vi "zmq_getsocketopt_binary.vi"(3 "error in":errorcluster, 4 "option":T1, 5 "socket in":refnum<class "Socket.lvclass">) -> (0 "error out":errorcluster, 1 "value":string, 2 "socket out":refnum<class "Socket.lvclass">)   [LabVIEW 2025, in "ZeroMQ.lvlib" / "Socket.lvclass"]
doc: "Query the value of <b>option</b> for the given <b>socket</b>.\n\nYou are responsible for selecting the correct polymorphic instance for the option you wish to query. Valid options of the binary type are: ZMQ_IDENTITY\n\nFurther API documentation: http://api.zeromq.org/3-2:zmq-getsockopt"
uses:
  Socket.lvclass
  socket_options.ctl
  Socket.lvclass/Socket.ctl
  ZeroMQ.lvlib
panel:
  out "len":u32
  # "ØMQ"
  # "labview"
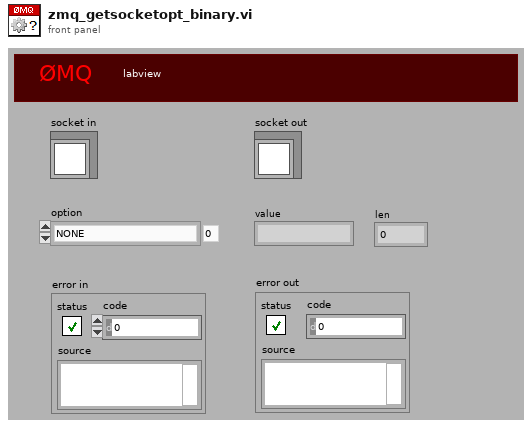
[diagram p1: front panel]
types:
  T1 = typedef "ZeroMQ.lvlib/socket_options.ctl" = enum8{"NONE", "ZMQ_HWM", "<2>", "ZMQ_SWAP", "ZMQ_AFFINITY", "ZMQ_ROUTING_ID", "ZMQ_SUBSCRIBE", "ZMQ_UNSUBSCRIBE", "ZMQ_RATE", "ZMQ_RECOVERY_IVL", "ZMQ_MCAST_LOOP", "ZMQ_SNDBUF", "ZMQ_RCVBUF", "ZMQ_RCVMORE", "ZMQ_FD", "ZMQ_EVENTS", "ZMQ_TYPE", "ZMQ_LINGER", "ZMQ_RECONNECT_IVL", "ZMQ_BACKLOG", "ZMQ_RECOVERY_IVL_MSEC", "ZMQ_RECONNECT_IVL_MAX", "ZMQ_MAXMSGSIZE", "ZMQ_SNDHWM", "ZMQ_RCVHWM", "ZMQ_MULTICAST_HOPS", "<26>", "ZMQ_RCVTIMEO", "ZMQ_SNDTIMEO", "<29>", "<30>", "ZMQ_IPV4ONLY", "ZMQ_LAST_ENDPOINT", "ZMQ_ROUTER_MANDATORY", "ZMQ_TCP_KEEPALIVE", "ZMQ_TCP_KEEPALIVE_CNT", "ZMQ_TCP_KEEPALIVE_IDLE", "ZMQ_TCP_KEEPALIVE_INTVL", "ZMQ_TCP_ACCEPT_FILTER", "ZMQ_IMMEDIATE", "ZMQ_XPUB_VERBOSE", "ZMQ_ROUTER_RAW", "ZMQ_IPV6", "ZMQ_MECHANISM", "ZMQ_PLAIN_SERVER", "ZMQ_PLAIN_USERNAME", "ZMQ_PLAIN_PASSWORD", "ZMQ_CURVE_SERVER", "ZMQ_CURVE_PUBLICKEY", "ZMQ_CURVE_SECRETKEY", "ZMQ_CURVE_SERVERKEY", "ZMQ_PROBE_ROUTER", "ZMQ_REQ_CORRELATE", "ZMQ_REQ_RELAXED", "ZMQ_CONFLATE", "ZMQ_ZAP_DOMAIN", "ZMQ_ROUTER_HANDOVER", "ZMQ_TOS", "ZMQ_IPC_FILTER_PID", "ZMQ_IPC_FILTER_UID", "ZMQ_IPC_FILTER_GID", "ZMQ_CONNECT_ROUTING_ID", "ZMQ_GSSAPI_SERVER", "ZMQ_GSSAPI_PRINCIPAL", "ZMQ_GSSAPI_SERVICE_PRINCIPAL", "ZMQ_GSSAPI_PLAINTEXT", "ZMQ_HANDSHAKE_IVL", "<67>", "ZMQ_SOCKS_PROXY", "ZMQ_XPUB_NODROP", "ZMQ_BLOCKY", "ZMQ_XPUB_MANUAL", "ZMQ_XPUB_WELCOME_MSG", "ZMQ_STREAM_NOTIFY", "ZMQ_INVERT_MATCHING", "ZMQ_HEARTBEAT_IVL", "ZMQ_HEARTBEAT_TTL", "ZMQ_HEARTBEAT_TIMEOUT", "ZMQ_XPUB_VERBOSER", "ZMQ_CONNECT_TIMEOUT", "ZMQ_TCP_MAXRT", "ZMQ_THREAD_SAFE", "<82>", "<83>", "ZMQ_MULTICAST_MAXTPDU", "ZMQ_VMCI_BUFFER_SIZE", "ZMQ_VMCI_BUFFER_MIN_SIZE", "ZMQ_VMCI_BUFFER_MAX_SIZE", "ZMQ_VMCI_CONNECT_TIMEOUT", "ZMQ_USE_FD", "ZMQ_GSSAPI_PRINCIPAL_NAMETYPE", "ZMQ_GSSAPI_SERVICE_PRINCIPAL_NAMETYPE", "ZMQ_BINDTODEVICE", "ZMQ_ZAP_ENFORCE_DOMAIN", "ZMQ_LOOPBACK_FASTPATH", "ZMQ_METADATA", "ZMQ_MULTICAST_LOOP", "ZMQ_ROUTER_NOTIFY"}
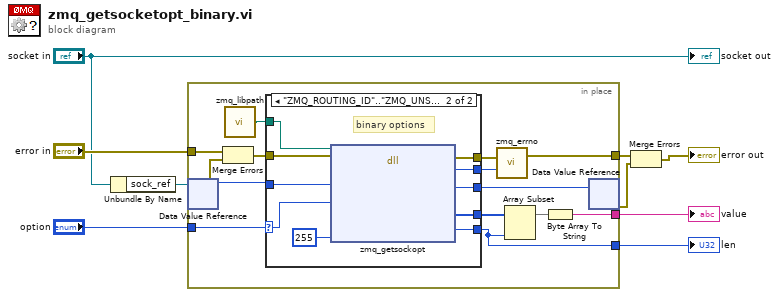
[diagram p0: block diagram]
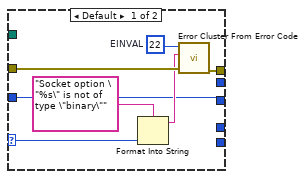
[diagram p2: hidden frame]
diagram:
  n1 = Unbundle By Name("socket in") -> ("sock_ref"=w3:refnum<data-value>)
  n2 = in-place {
    in-place-border: [w21] -> w9
    in-place-border: "error in" -> [w20]
    in-place-border: "option" -> [w19]
    in-place-border: [w10] -> w6
    in-place-border: [w11] -> w5
    n3 = in-place-dvr #1(w3) -> (w17:u64, w13:errorcluster)
    n4 = Merge Errors(w20, w13) -> (w14:errorcluster)
    n5 = call "zmq_libpath.vi"() -> ("path"=w15:path)  [unwired: 1 in]
    n6 = case shown="\"ZMQ_ROUTING_ID\"..\"ZMQ_UNSUBSCRIBE\", \"ZMQ_LAST_ENDPOINT\", \"ZMQ_TCP_ACCEPT_FILTER\", \"ZMQ_PLAIN_USERNAME\", \"ZMQ_PLAIN_PASSWORD\", \"ZMQ_CURVE_PUBLICKEY\"..\"ZMQ_CURVE_SERVERKEY\", \"ZMQ_ZAP_DOMAIN\", \"ZMQ_CONNECT_ROUTING_ID\", \"ZMQ_GSSAPI_PRINCIPAL\", \"ZMQ_GSSAPI_SERVICE_PRINCIPAL\", \"ZMQ_SOCKS_PROXY\", \"ZMQ_XPUB_WELCOME_MSG\", \"ZMQ_BINDTODEVICE\", \"ZMQ_METADATA\"" w19 {
      selector: w19 -> [w27 w38]
      tunnel: [w30 w40] -> w23
      tunnel: [_ w39] -> w22
      tunnel: w14 -> [w28 w36]
      tunnel: [_ w35] -> w18
      tunnel: [_ w34] -> w11
      tunnel: w17 -> [w24 w33]
      tunnel: [w24 w32] -> w16
      tunnel: w15 -> [_ w31]
      frame Default {
        w29 = 22  # EINVAL
        n7 = Format Into String(format string="Socket option \"%s\" is not of type \"binary\"", w27) -> (resulting string=w25:string)  [unwired: 2 in, 1 out]
        n8 = call <vilib>:"Error Cluster From Error Code.vi"("error in (no error)"=w28, "error message (\"\")"=w25, "error code (0)"=w29) -> ("error out"=w30:errorcluster)  [unwired: 6 in]
      }
      frame "ZMQ_ROUTING_ID".."ZMQ_UNSUBSCRIBE", "ZMQ_LAST_ENDPOINT", "ZMQ_TCP_ACCEPT_FILTER", "ZMQ_PLAIN_USERNAME", "ZMQ_PLAIN_PASSWORD", "ZMQ_CURVE_PUBLICKEY".."ZMQ_CURVE_SERVERKEY", "ZMQ_ZAP_DOMAIN", "ZMQ_CONNECT_ROUTING_ID", "ZMQ_GSSAPI_PRINCIPAL", "ZMQ_GSSAPI_SERVICE_PRINCIPAL", "ZMQ_SOCKS_PROXY", "ZMQ_XPUB_WELCOME_MSG", "ZMQ_BINDTODEVICE", "ZMQ_METADATA" {
        # "binary options"
        n9 = dll-call lib="C:/git/ZA/src/zeromq/lib/win32/libzmq-v143-mt-4_3_6.dll" fn="zmq_getsockopt" ("zmq_labview.dll:lvzmq_getsockopt")(path in=w31, error in=w36, "socket"=w33, "option"=w38, "len"=u32 255) -> (error out=w40:errorcluster, "return type"=w39:i32, "socket"=w32:u64, "data"=w35:u8[], "len"=w34:u32)  [unwired: 3 in, 1 out]
      }
    }
    n10 = call "zmq_errno.vi"("retval"=w22, "error in"=w23) -> ("error out"=w21:errorcluster)  [unwired: 1 out]
    n11 = Array Subset(array=w18, length=w11) -> (w12:u8[])  [unwired: 1 in]
    n12 = Byte Array To String(unsigned byte array=w12) -> (string=w10:string)
    n13 = in-place-dvr #1(w16) -> (w1:errorcluster)  [unwired: 1 out]
  }
  "value" <- w6
  "len" <- w5
  n14 = Merge Errors(w9, w1) -> (→"error out":errorcluster)
  "socket out" <- "socket in"
